vi "MHP30 State Machine.vi"() -> ()   [LabVIEW 2019]
panel:
  in  "Preset":i32(listbox)
  in  "Settings":i32(listbox)
  out "Mode":i32(listbox)
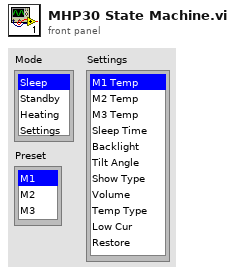
[diagram p1: front panel]
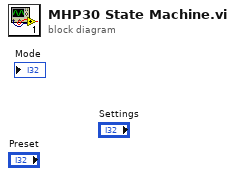
[diagram p0: block diagram]
diagram:
